vi "nanostage-main-quick-check-vis.vi"() -> ()   [LabVIEW 2015]
panel:
  out "error":bool
  out "error message":string
  out "moving":bool
  in  "setValues":dbl[](array[numeric])
  out "position-z":dbl
  out "position-y":dbl
  out "position-x":dbl
  in  "stop":bool
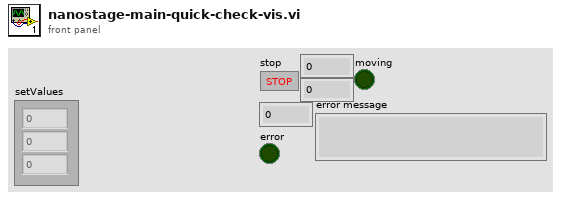
[diagram p1: front panel]
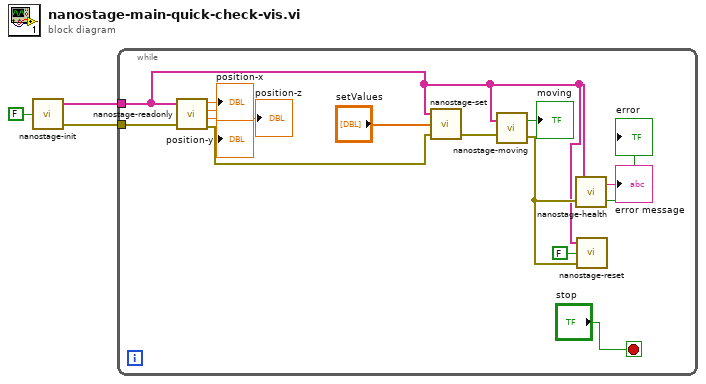
[diagram p0: block diagram]
diagram:
  n1 = call "nanostage-init.vi"("Perform autozero?"=FALSE) -> ("error out"=w3:errorcluster, "All conn. axes"=w2:string[])  [unwired: 3 in]
  n2 = while {
    tunnel: w3 -> [w16]
    tunnel: w2 -> [w5]
    stop <- "stop" stop-if-true
    n3 = call "nanostage-readonly.vi"("error in"=w16, "Axes to move"=w5) -> ("error out"=w11:errorcluster, "position-z"=→"position-z":dbl, "position-y"=→"position-y":dbl, "position-x"=→"position-x":dbl)  [unwired: 2 in]
    n4 = call "nanostage-set.vi"("error in"=w11, "setValues"="setValues", "Axes to move"=w5) -> ("error out"=w10:errorcluster)  [unwired: 1 in, 1 out]
    n5 = call "nanostage-moving.vi"("error in"=w10, "Axes to query"=w5) -> ("error out"=w6:errorcluster, "moving"=→"moving":bool)
    n6 = call "nanostage-health.vi"("error in"=w6, "All conn. axes"=w5) -> ("error"=→"error":bool, "error message"=→"error message":string)
    n7 = call "nanostage-reset.vi"("error in"=w6, "reset stage"=FALSE, "All conn. axes"=w5) -> ()  [unwired: 1 in, 2 out]
  }
